vi "Write DAQ Params.vi"(10 "DAQ Params":T1, 11 "Template in":refnum<class "Template.lvclass">) -> (3 "Template out":refnum<class "Template.lvclass">)   [LabVIEW 2020, in "Template.lvlib" / "Template.lvclass"]
uses:
  Template.lvclass
  typedefs/daq params.ctl
  Template.lvclass/Template.ctl
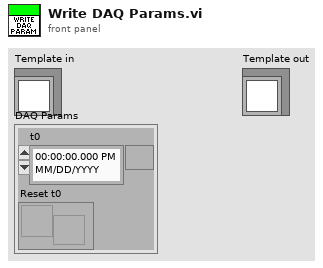
[diagram p1: front panel]
types:
  T1 = typedef "Template.lvlib/Template.lvclass/daq params.ctl" = cluster{"t0":timestamp, "Reset t0":refnum<notifier>}
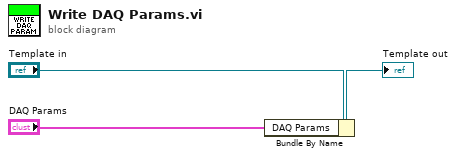
[diagram p0: block diagram]
diagram:
  n1 = Bundle By Name(cluster="Template in", "DAQ Params"="DAQ Params") -> (→"Template out":refnum<class "Template.lvclass">)
